vi "Fetch gRPC from Map.vi"(7 "gRPC Server Class type":refnum<class "ServiceBase.lvclass">, 8 "error in (no error)":errorcluster, 11 "Plugin Manager in":refnum<class "CIFPluginManager.lvclass">) -> (0 "error out":errorcluster, 2 "gRPC Server Class out":refnum<class "ServiceBase.lvclass">, 3 "Plugin Manager out":refnum<class "CIFPluginManager.lvclass">)   [LabVIEW 2021, in "CIFPluginManager.lvclass"]
uses:
  CIFPluginManager.lvclass
  <vilib>/gRPC/LabVIEW gRPC Servicer/ServiceBase/ServiceBase.lvclass
  <vilib>/CIF Foundation/CIF Core/CIFCore/Common/Typedef/Errors.ctl
  CIFPluginManager.lvclass/CIFPluginManager.ctl
  <vilib>/CIF Foundation/CIF Utilities/Errors/Append Error Location.vi
  <vilib>/CIF Foundation/CIF Core/CIFCore/Common/CIFCoreCommon.lvlib
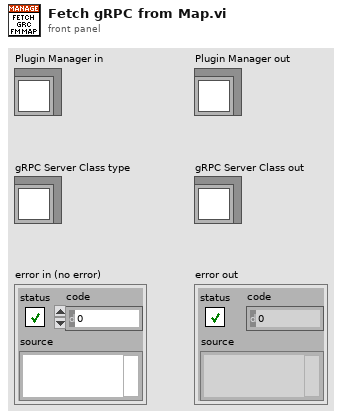
[diagram p1: front panel]
types:
  T1 = typedef "CIFCoreCommon.lvlib/Errors.ctl" = enum16{"Invalid Clock ID", "Long Sleep", "gRPC Server Not Found", "Config Parse", "Timestamp Wrap", "Delayed Execution", "Duplicate Channel", "Missing Channel", "Incorrect Type", "Flatten Error", "Unflatten Data", "Unique Name", "Plugin Not Found", "Plugin Type Not Found", "Plugin Version Not Found", "Manager Not Found", "Numerical Issue", "Time Jump", "Clock ID Match", "Channel Length", "Plugin Connection", "gRPC Server Connection", "PPL Name Match", "Build", "Config Log Parse", "Plugin Load", "UI Subpanel Load", "Python Name", "Invalid Name", "Unable to Change Ch Buffer", "Failed Kill", "Failed SysExec", "Function Not Implemented", "Load Timeout"}
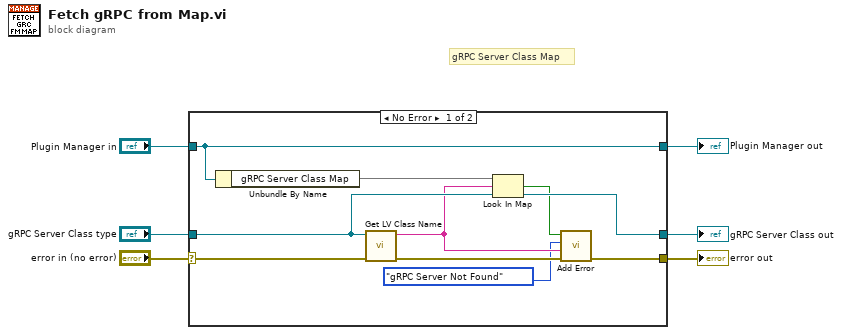
[diagram p0: block diagram]
diagram:
  # "gRPC Server Class Map"
  n1 = case shown="No Error" "error in (no error)" {
    selector: "error in (no error)" -> [w16 w18]
    tunnel: [w12 w18] -> w2
    tunnel: [w8 w19] -> w4
    tunnel: "Plugin Manager in" -> [w8 w19]
    tunnel: "gRPC Server Class type" -> [w14 w17]
    tunnel: [w15 w17] -> w6
    frame No Error {
      n2 = Unbundle By Name(w8) -> ("gRPC Server Class Map"=w7:map{string, refnum<class "ServiceBase.lvclass">})
      n3 = call <vilib>:"Get LV Class Name.vi"("error in (no error)"=w16, "object"=w14) -> ("error out"=w13:errorcluster, "class name"=w11:string)  [unwired: 8 in]
      n4 = Look In Map(map=w7, key=w11, default value=w14) -> (key not found?=w10:bool, value=w15:refnum<class "ServiceBase.lvclass">)
      n5 = call <vilib>:"Add Error.vi"("error in (no error)"=w13, "String to Append"=w11, "Error"=Errors."gRPC Server Not Found", "Insert Error"=w10) -> ("error out"=w12:errorcluster)  [unwired: 7 in]
    }
    frame Error {
    }
  }
  "error out" <- w2
  "Plugin Manager out" <- w4
  "gRPC Server Class out" <- w6
